vi "Fit VI window to Visible Content.vi"(4 "error in (no error)":errorcluster, 6 "border spacing (2 px)":i32=2, 7 "VI Ref (calling VI)":refnum<vi>) -> (0 "error out":errorcluster, 3 "dup VI Ref":refnum<vi>)   [LabVIEW 2017]
doc: "Resizes and centres the VI window around the visible front panel objects, adding the configured border spacing in pixels. With no VI reference wired it operates on the calling VI."
panel:
  # "Fit VI window to Content.vi\n\nFits a VI's front panel window to its FP Contents.\n\nPlease visit http://www.OpenG.org to learn about the\nOpen Source LabVIEW software movement.\n\nNOTICE -- YOU MUST LEAVE THIS NOTICE IN PLACE.  PER THE TERMS OF THE LICENSE BELOW, YOU MAY SUBLICENSE THIS SOFTWARE \nIN ANY WAY THAT DOES NOT CONFLICT WITH THIS LICENSE.\n\n### BSD License (http://www.opensource.org/licenses/bsd-license.php) Begin ###\n \nCopyright (c) 2002-2004, Jim Kring <jim@jimkring.com>\nCopyright (c) 2002, Cal-Bay Systems, Inc. <info@calbay.com>\n\nAll rights reserved.\n\nRedistribution and use in source and binary forms, with or without modification, are permitted provided that the following conditions are met:\n\n    * Redistributions of source code must retain the above copyright notice, this list of conditions and the following disclaimer.\n    * Redistributions in binary form must reproduce the above copyright notice, this list of conditions and the following disclaimer in the \n       documentation and/or other materials provided with the distribution.\n    * Neither the name of SciWare, James Kring, Inc., nor the names of its contributors may be used to endorse or promote products derived \n       from this software without specific prior written permission.\n\nTHIS SOFTWARE IS PROVIDED BY THE COPYRIGHT HOLDERS AND CONTRIBUTORS \"AS IS\" AND ANY EXPRESS OR IMPLIED WARRANTIES, \nINCLUDING, BUT NOT LIMITED TO, THE IMPLIED WARRANTIES OF MERCHANTABILITY AND FITNESS FOR A PARTICULAR PURPOSE ARE \nDISCLAIMED. IN NO EVENT SHALL THE COPYRIGHT OWNER OR CONTRIBUTORS BE LIABLE FOR ANY DIRECT, INDIRECT, INCIDENTAL,\n SPECIAL, EXEMPLARY, OR CONSEQUENTIAL DAMAGES (INCLUDING, BUT NOT LIMITED TO, PROCUREMENT OF SUBSTITUTE GOODS OR \nSERVICES; LOSS OF USE, DATA, OR PROFITS; OR BUSINESS INTERRUPTION) HOWEVER CAUSED AND ON ANY THEORY OF LIABILITY, \nWHETHER IN CONTRACT, STRICT LIABILITY, OR TORT (INCLUDING NEGLIGENCE OR OTHERWISE) ARISING IN ANY WAY OUT OF THE USE \nOF THIS SOFTWARE, EVEN IF ADVISED OF THE POSSIBILITY OF SUCH DAMAGE.\n\n### BSD License End ###"
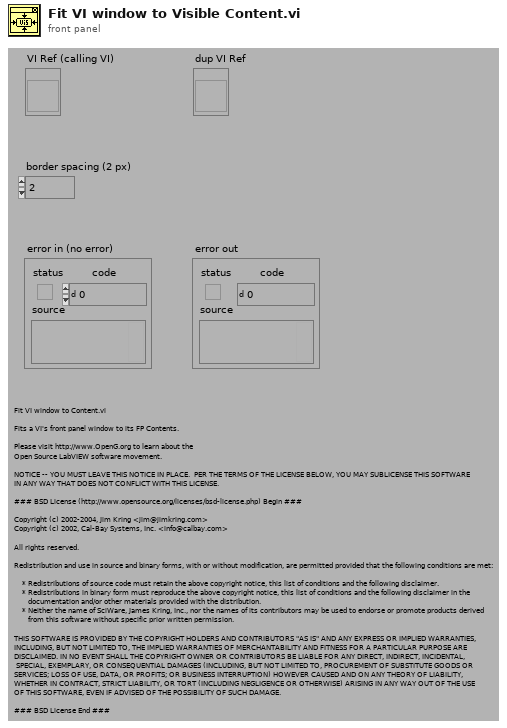
[diagram p1: front panel]
types:
  T1 = typedef "LVRectTypeDef.ctl" = cluster{"Left":i16, "Top":i16, "Right":i16, "Bottom":i16}
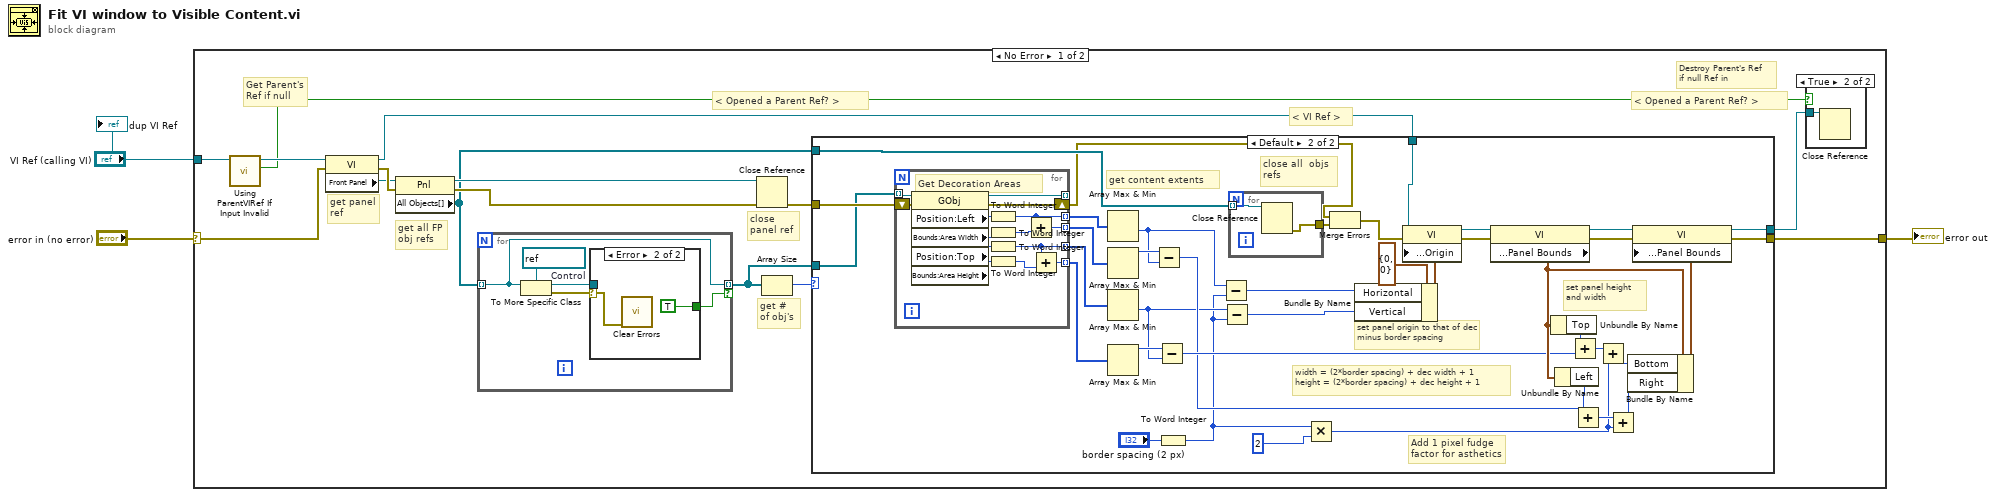
[diagram p0: block diagram]
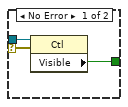
[diagram p2: hidden frame]
diagram:
  n1 = case shown="No Error" "error in (no error)" {
    selector: "error in (no error)" -> [w8 w87]
    tunnel: [w12 w87] -> w3
    tunnel: "VI Ref (calling VI)" -> [w9 _]
    frame No Error {
      # "< Opened a Parent Ref? >"
      # "< Opened a Parent Ref? >"
      # "Destroy Parent's Ref\nif null Ref in"
      # "Get Parent's\nRef if null"
      # "get # of obj's"
      # "get panel ref"
      # "get all FP obj refs"
      # "close panel ref"
      # "< VI Ref >"
      n2 = call "Using ParentVIRef If Input Invalid.vi"("VI Ref (calling VI)"=w9) -> ("Using Parent Ref(Need to Destroy)"=w4:bool, "VI Ref"=w5:refnum<vi>)  [unwired: 5 in]
      n3 = property on="Property Node" class="VI"(reference=w5, error in=w8) -> (reference out=w18:refnum<vi>, error out=w16:errorcluster, "Front Panel"=w14:refnum<vi>)
      n4 = property on="Property Node" class="Pnl"(reference=w14, error in=w16) -> (reference out=w17:refnum<vi>, error out=w15:errorcluster, "All Objects[]"=w7:refnum<vi>[])
      n5 = for {
        tunnel: [w19] -> w6 mode=indexing if=w20
        tunnel: w7 -> [w19] mode=indexing
        w22 = refnum<vi> refnum  # Control
        n6 = To More Specific Class(target class=w22, reference=w19) -> (specific class reference=w23:refnum<vi>, error out=w21:errorcluster)  [unwired: 1 in]
        n7 = case shown="Error" w21 {
          selector: w21 -> [w25 w27]
          tunnel: w23 -> [w26 _]
          tunnel: [w24 TRUE ("Visible")] -> w20
          frame No Error {
            n8 = property class="Ctl"(reference=w26, error in=w25) -> ("Visible"=w24:bool)  [unwired: 2 out]
          }
          frame Error {
            n9 = call <vilib>:"Clear Errors.vi"("error in (no error)"=w27) -> ()  [unwired: 5 in, 2 out]
          }
        }
      }
      n10 = Close Reference(reference=w17, error in (no error)=w15) -> (error out=w13:errorcluster)
      n11 = Array Size(array=w6) -> (size(s)=w11:i32)
      n12 = case shown="Default" w11 {
        tunnel: w18 -> [w31 w68]
        tunnel: w13 -> [w30 w55]
        tunnel: [w30 w50] -> w12
        tunnel: [w31 w49] -> w10
        tunnel: w7 -> [_ w35]
        tunnel: w6 -> [_ w34]
        frame 0 {
          # "do nothing if no objects"
        }
        frame Default {
          # "width = (2*border spacing) + dec width + 1\nheight = (2*border spacing) + dec height + 1"
          # "set panel height and width"
          # "set panel origin to that of dec minus border spacing"
          # "close all  objs refs"
          # "get content extents"
          # "Add 1 pixel fudge factor for asthetics"
          n13 = for {
            tunnel: w34 -> [w86] mode=indexing
            shift-right: [w84] -> w32
            shift-left: w55 -> [w85]
            tunnel: [w83] -> _ mode=indexing
            tunnel: [w79] -> w47 mode=indexing
            tunnel: [w81] -> w46 mode=indexing
            tunnel: [w75] -> w45 mode=indexing
            tunnel: [w80] -> w44 mode=indexing
            # "Get Decoration Areas"
            n14 = property class="GObj"(reference=w86, error in=w85) -> (reference out=w83:refnum<vi>, error out=w84:errorcluster, "Position:Left"=w82:i32, "Bounds:Area Width"=w78:u32, "Position:Top"=w76:i32, "Bounds:Area Height"=w74:u32)
            n15 = To Word Integer(number=w82) -> (16bit integer=w79:i16)
            n16 = To Word Integer(number=w78) -> (16bit integer=w77:i16)
            n17 = To Word Integer(number=w76) -> (16bit integer=w75:i16)
            n18 = To Word Integer(number=w74) -> (16bit integer=w73:i16)
            n19 = Add(x=w79, y=w77) -> (x+y=w81:i16)
            n20 = Add(x=w75, y=w73) -> (x+y=w80:i16)
          }
          n21 = Array Max & Min(array=w47) -> (min value=w38:i16)  [unwired: 3 out]
          n22 = Array Max & Min(array=w46) -> (max value=w41:i16)  [unwired: 3 out]
          n23 = Array Max & Min(array=w45) -> (min value=w39:i16)  [unwired: 3 out]
          n24 = Array Max & Min(array=w44) -> (max value=w43:i16)  [unwired: 3 out]
          n25 = Subtract(x=w41, y=w38) -> (x-y=w40:i16)
          n26 = Subtract(x=w43, y=w39) -> (x-y=w42:i16)
          n27 = To Word Integer(number="border spacing (2 px)") -> (16bit integer=w36:i16)
          n28 = Subtract(x=w38, y=w36) -> (x-y=w58:i16)
          n29 = Subtract(x=w39, y=w36) -> (x-y=w59:i16)
          n30 = for {
            tunnel: w35 -> [w71] mode=indexing
            tunnel: [w72] -> w37
            n31 = Close Reference(reference=w71) -> (error out=w72:errorcluster)  [unwired: 1 in]
          }
          n32 = Multiply(x=w36, y=i16 2) -> (x*y=w48:i16)
          n33 = Merge Errors(w32, w37) -> (w33:errorcluster)
          n34 = Bundle By Name(cluster=cluster{"Horizontal":i16, "Vertical":i16} {"Horizontal"=0, "Vertical"=0} ("Front Panel Window:Origin"), "Horizontal"=w58, "Vertical"=w59) -> (w56:cluster{"Horizontal":i16, "Vertical":i16})
          n35 = property on="Property Node" class="VI"(reference=w68, error in=w33, "Front Panel Window:Origin"=w56) -> (reference out=w69:refnum<vi>, error out=w52:errorcluster)
          n36 = property on="Property Node" class="VI"(reference=w69, error in=w52) -> (reference out=w70:refnum<vi>, error out=w51:errorcluster, "Front Panel Window:Panel Bounds"=w60:T1)
          n37 = Unbundle By Name(w60) -> ("Top"=w61:i16)
          n38 = Unbundle By Name(w60) -> ("Left"=w62:i16)
          n39 = Add(x=w61, y=w42) -> (x+y=w66:i16)
          n40 = Add(x=w62, y=w40) -> (x+y=w64:i16)
          n41 = Add(x=w66, y=w48) -> (x+y=w67:i16)
          n42 = Add(x=w64, y=w48) -> (x+y=w65:i16)
          n43 = Bundle By Name(cluster=w60, "Bottom"=w67, "Right"=w65) -> (w63:T1)
          n44 = property on="Property Node" class="VI"(reference=w70, error in=w51, "Front Panel Window:Panel Bounds"=w63) -> (reference out=w49:refnum<vi>, error out=w50:errorcluster)
        }
      }
      n45 = case shown="True" w4 {
        tunnel: w10 -> [_ w29]
        frame False {
        }
        frame True {
          n46 = Close Reference(reference=w29) -> ()  [unwired: 1 in, 1 out]
        }
      }
    }
    frame Error {
    }
  }
  "error out" <- w3
  "dup VI Ref" <- "VI Ref (calling VI)"
